vi "Write SCH Secondary Config Parameters to FPGA.vi"(8 "error in (no error)":errorcluster, 10 "FPGA Configuration Values":T1={"Ln2 Filter Size"=10, "CoWound Volt Limit"=4000000.0, "CoWound Tick Limit"=0, "DAQ Cycle Ticks"=4000000, "Co-Wound Asymmetry Factor"=0.0002000033855438, "Co-Wound Scale Factor"=0.2000122070312, "# Consecutive Zeros Fault"=2304, "Digitize Convert Ticks"=0, "Digitize Reset Ticks"=4000000, "Convert Clock Ticks"=1000000, "Digitize Read Delay Ticks"=4096, "Digitize # Bits"=256, "Low Current (kA)"=38.14697265625, "Low Current Ticks"=6, "Low Current Delay Factor"=1, "Cold Mass Scale Factor"=59.988, "Current Scale Factor"=2.0} {"Current Scale Factor" format="%_6g"; "Co-Wound Asymmetry Factor" format="%.8g"}, 11 "Refnum in":T2) -> (0 "error out":errorcluster, 3 "Refnum out":T2)   [LabVIEW 2020]
doc: "Author: Scott Hannahs <sth@magnet.fsu.edu>\nCopyright 2018 Florida State University, All rights reserved."
uses:
  RT Controls/FPGA SCH Secondary Digitizer Ref.ctl
  SCH Data Controls/FPGA Secondary Configure Parameters.ctl
  <vilib>/Utility/error.llb/Error Cluster From Error Code.vi
  <vilib>/rvi/errors/niLvFpgaAdjustHostInterfaceError.vi
  <vilib>/rvi/interface/nirviReadWriteControl/nirviReadWriteControl.xnode
  NiFpgaLv.dll
  <vilib>/rvi/interface/Simulation/niFpgaSimulationCallBeginRW.vi
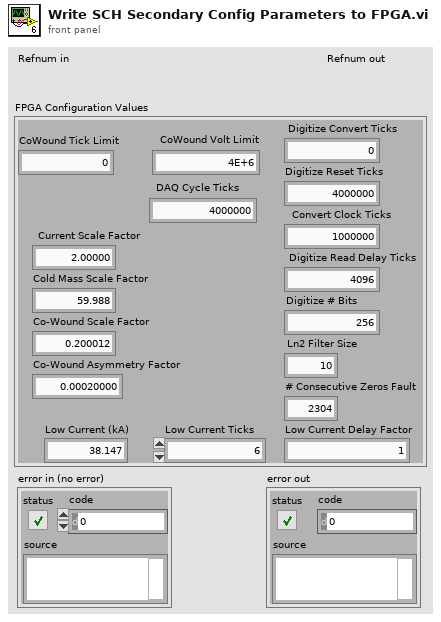
[diagram p1: front panel]
types:
  T1 = typedef "FPGA Secondary Configure Parameters.ctl" = cluster{"Ln2 Filter Size":i16, "CoWound Volt Limit":dbl, "CoWound Tick Limit":u32, "DAQ Cycle Ticks":u32, "Co-Wound Asymmetry Factor":dbl, "Co-Wound Scale Factor":dbl, "# Consecutive Zeros Fault":i16, "Digitize Convert Ticks":u32, "Digitize Reset Ticks":u32, "Convert Clock Ticks":u32, "Digitize Read Delay Ticks":u32, "Digitize # Bits":u32, "Low Current (kA)":dbl, "Low Current Ticks":u32, "Low Current Delay Factor":u16, "Cold Mass Scale Factor":dbl, "Current Scale Factor":dbl}
  T2 = typedef "FPGA SCH Secondary Digitizer Ref.ctl" = refnum<k20>
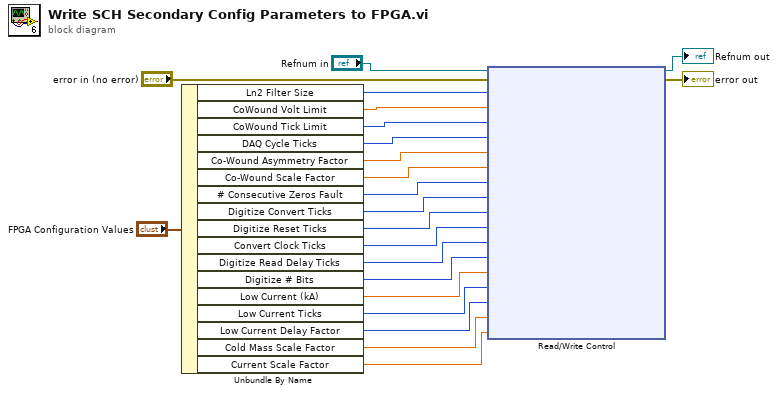
[diagram p0: block diagram]
diagram:
  n1 = Unbundle By Name("FPGA Configuration Values") -> ("Ln2 Filter Size"=w17:i16, "CoWound Volt Limit"=w16:dbl, "CoWound Tick Limit"=w15:u32, "DAQ Cycle Ticks"=w14:u32, "Co-Wound Asymmetry Factor"=w13:dbl, "Co-Wound Scale Factor"=w12:dbl, "# Consecutive Zeros Fault"=w11:i16, "Digitize Convert Ticks"=w10:u32, "Digitize Reset Ticks"=w9:u32, "Convert Clock Ticks"=w8:u32, "Digitize Read Delay Ticks"=w7:u32, "Digitize # Bits"=w6:u32, "Low Current (kA)"=w5:dbl, "Low Current Ticks"=w4:u32, "Low Current Delay Factor"=w3:u16, "Cold Mass Scale Factor"=w2:dbl, "Current Scale Factor"=w1:dbl)
  n2 = xnode "Read/Write Control"("FPGA VI Reference In"="Refnum in", "error in"="error in (no error)", "Ln2 Filter Size"=w17, "CoWound Volt Limit"=w16, "CoWound Tick Limit"=w15, "DAQ Cycle Ticks"=w14, "Co-Wound Asymmetry Factor"=w13, "Co-Wound Scale Factor"=w12, "# Consecutive Zeros Fault"=w11, "Digitize Convert Ticks"=w10, "Digitize Reset Ticks"=w9, "Convert Clock Ticks"=w8, "Digitize Read Delay Ticks"=w7, "Digitize # Bits"=w6, "Low Current (kA)"=w5, "Low Current Ticks"=w4, "Low Current Delay Factor"=w3, "Cold Mass Scale Factor"=w2, "Current Scale Factor"=w1) -> ("FPGA VI Reference Out"=→"Refnum out":T2, "error out"=→"error out":errorcluster)
